vi "Termination Character Parser.vi"(11 "Termination Char":T1=enum."\\r\\n") -> (3 "String":string)   [LabVIEW 2014, in "Serial Base.lvclass"]
uses:
  Serial Base.lvclass
  Termination Character--enum.ctl
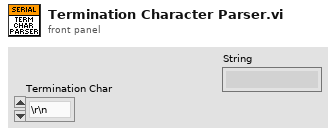
[diagram p1: front panel]
types:
  T1 = typedef "Serial Base.lvclass/Termination Character--enum.ctl" = enum16{"none", "\\r\\n", "\\r", "\\n"}
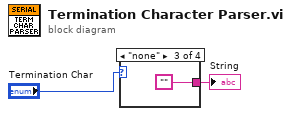
[diagram p0: block diagram]
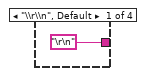
[diagram p2: hidden frame]
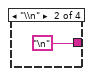
[diagram p3: hidden frame]
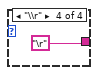
[diagram p4: hidden frame]
diagram:
  n1 = case shown="\"none\"" "Termination Char" {
    tunnel: ["\r\n" "\n" "" "\r"] -> w1
    frame "\\r\\n", Default {
    }
    frame "\\n" {
    }
    frame "none" {
    }
    frame "\\r" {
    }
  }
  "String" <- w1
